vi "GeneratePositionResponsePWM.vi"(10 "PWM Width (s)":dbl format="%#_13g", 11 "Position (um)":dbl) -> (2 "Position rounded down (mm)":i32, 3 "PWM Signal":bool)   [LabVIEW 2014]
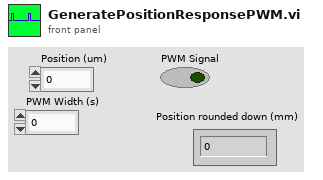
[diagram p1: front panel]
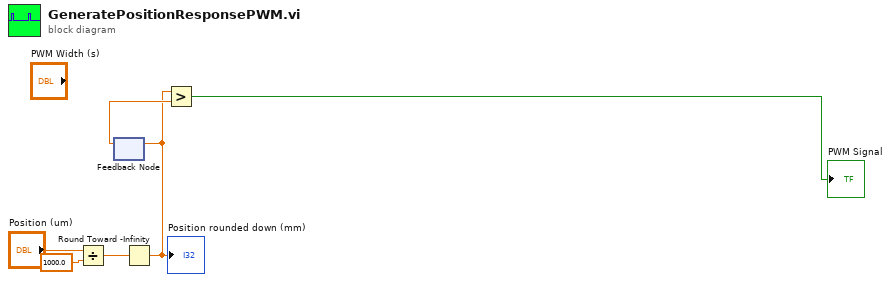
[diagram p0: block diagram]
diagram:
  n1 = Divide ("Divide 2")(x="Position (um)", y=1000.0 ("Constant")) -> (x/y=w3:dbl)
  n2 = feedback #1() -> (w6:dbl)  [unwired: 1 in]
  n3 = Round Toward -Infinity(1:w3) -> (0:w5:dbl)
  "Position rounded down (mm)" <- w5
  n4 = feedback-in #1(w5) -> ()
  n5 = Greater? ("Greater? 2")(x=w5, y=w6) -> (0:→"PWM Signal":bool)
